vi "SF2_Send_Notifier.vi"(9 "Data":variant, 11 "SF2 Action":T1) -> ()   [LabVIEW 2016]
uses:
  SF2_ActionTypeDef.ctl
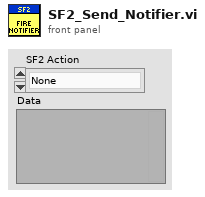
[diagram p1: front panel]
types:
  T1 = typedef "SF2_ActionTypeDef.ctl" = enum16{"None", "Halt", "Reset Buffer"}
  T2 = typedef "SF2_NotifyPacketTypeDef.ctl" = cluster{"SF2 Action":T1, "Data":variant}
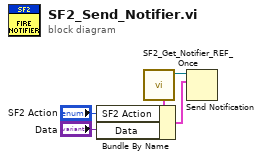
[diagram p0: block diagram]
diagram:
  n1 = call "SF2_Get_Notifier_REF_Once.vi"() -> ("notifier ref out"=w5:refnum<notifier>, "notification"=w4:T2)  [unwired: 10 in]
  n2 = Bundle By Name(cluster=w4, "SF2 Action"="SF2 Action", "Data"="Data") -> (w3:T2)
  n3 = Send Notification(notification=w3, notifier=w5) -> ()  [unwired: 1 in, 2 out]
